vi "HumanGlobal.vi"() -> ()   [LabVIEW 2020]
panel:
  out "RumbleToggle":bool
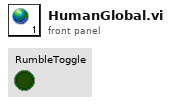
[diagram p1: front panel]
diagram:
